vi "Get Sender.vi"(11 "Msg Strategy in":refnum<class "Msg Strategy.lvclass">) -> (2 "Sender":refnum<class "Sender.lvclass">)   [LabVIEW 2021, in "jettl.lvlib" / "Msg Strategy.lvclass"]
uses:
  Msg Strategy.lvclass
  Sender/Sender/Sender.lvclass
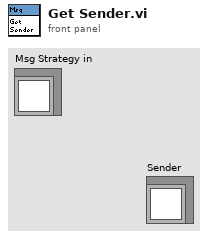
[diagram p1: front panel]
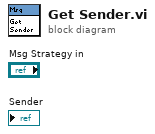
[diagram p0: block diagram]
diagram:
